vi "RP IV pattern write.vi"(4 "no bram":bool, 8 "Error In":errorcluster, 9 "Waveform parameters":T1={"Start magnitude"=1000.0, "Magnitude increment"=1000.0, "Number of pulses"=8, "Baseline length"=480, "Ramp length"=32, "Top  length"=480, "Threshold "=3000, "Processing delay"=240}, 11 "connection ID":refnum<k5>) -> (0 "Error Out":errorcluster, 3 "connection ID out":refnum<k5>, 5 "Waveform Graph":i16[](graph))   [LabVIEW 2016]
uses:
  Waform generation/Waveform parameters.ctl
  RP Command.ctl
  RP Write Command TCP.vi
panel:
  in  "Pattern":enum16{"Sine ramp", "Square"}(ring)
  out "Waveform length":u32=2048
  in  "Config offset":u64=20
  out "Step length":u32=2048
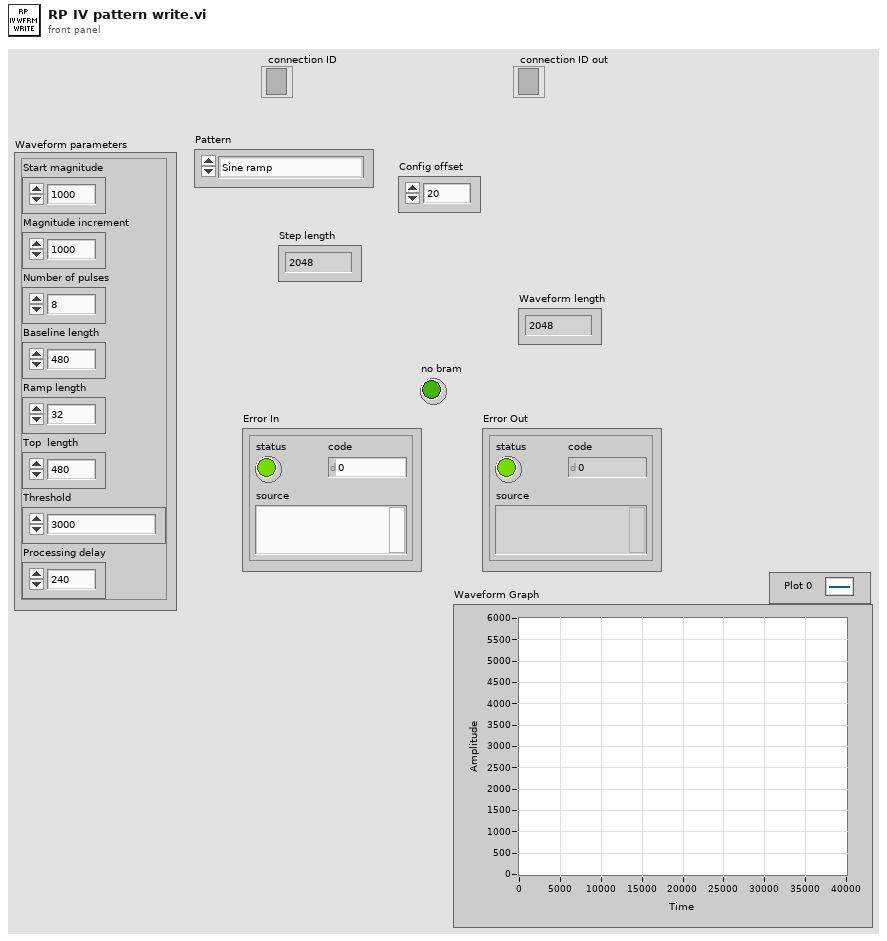
[diagram p1: front panel]
types:
  T1 = typedef "Waveform parameters.ctl" = cluster{"Start magnitude":dbl, "Magnitude increment":dbl, "Number of pulses":i32, "Baseline length":i32, "Ramp length":i32, "Top  length":i32, "Threshold ":i32, "Processing delay":u16}
  T2 = typedef "RP Command.ctl" = enum16{"Reset", "Read IDN", "Stop server", "Get status", "Get temperature", "Connect client", "Arm", "Software trigger", "Get whole buffer", "Get chunk", "System call", "Get config", "Set config", "Recieve data", "Recieve Calibartion", "Transmit data"}
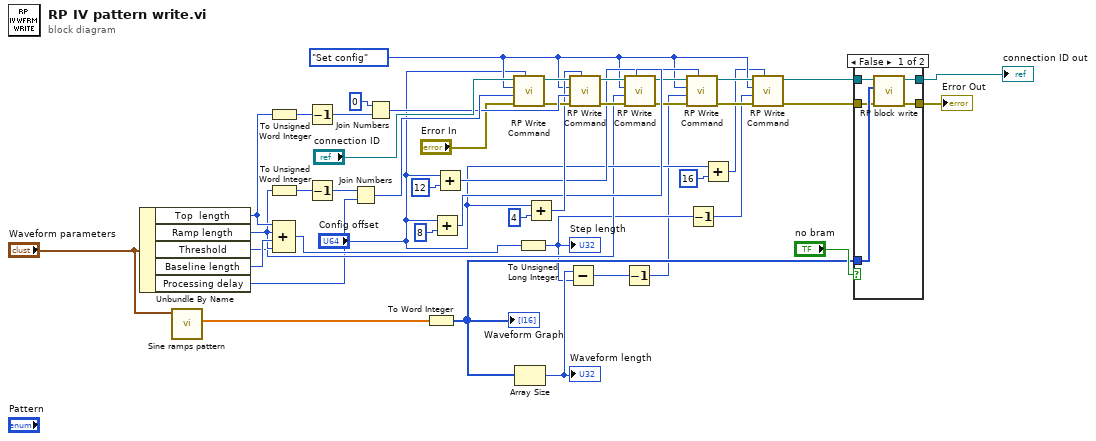
[diagram p0: block diagram]
diagram:
  w27 = RP_Command."Set config" ("Command number")
  n1 = Unbundle By Name("Waveform parameters") -> ("Top  length"=w16:i32, "Ramp length"=w14:i32, "Threshold"=w9:i32, "Baseline length"=w15:i32, "Processing delay"=w5:u16)
  n2 = call "Sine ramps pattern.vi"("Waveform parameters 2"="Waveform parameters") -> ("Waveform"=w17:dbl[])  [unwired: 8 in, 1 out]
  n3 = To Unsigned Word Integer(number=w16) -> (unsigned 16bit integer=w10:u16)
  n4 = To Unsigned Word Integer(number=w14) -> (unsigned 16bit integer=w11:u16)
  n5 = Compound Arithmetic op=ADD(w16, w14, w15, w14) -> (w7:i32)
  n6 = Decrement(x=w10) -> (x-1=w3:u16)
  n7 = Decrement(x=w11) -> (x-1=w4:u16)
  n8 = Join Numbers(hi=w4, lo=w5) -> ((hi.lo)=w45:u32)
  n9 = Join Numbers(hi=u16 0, lo=w3) -> ((hi.lo)=w42:u32)
  n10 = To Word Integer(number=w17) -> (16bit integer=w13:i16[])
  "Waveform Graph" <- w13
  n11 = Add(x="Config offset", y=u64 8) -> (x+y=w34:u64)
  n12 = Add(x="Config offset", y=u64 12) -> (x+y=w30:u64)
  n13 = call-poly "RP Write Command.vi"("Config offset"="Config offset", "Error In"="Error In", "Command payload"=w45, "Command number"=w27, "connection ID"="connection ID") -> ("Error Out"=w41:errorcluster, "connection ID out"=w44:refnum<k5>)  [unwired: 4 in, 1 out]
  n14 = Array Size(array=w13) -> (size(s)=w12:i32)
  "Waveform length" <- w12
  n15 = To Unsigned Long Integer(number=w7) -> (unsigned 32bit integer=w6:u32)
  "Step length" <- w6
  n16 = Add(x="Config offset", y=u64 4) -> (x+y=w38:u64)
  n17 = Subtract(x=w12, y=w6) -> (x-y=w8:u32)
  n18 = call-poly "RP Write Command.vi"("Config offset"=w38, "Error In"=w41, "Command payload"=w42, "Command number"=w27, "connection ID"=w44) -> ("Error Out"=w36:errorcluster, "connection ID out"=w37:refnum<k5>)  [unwired: 4 in, 1 out]
  n19 = Decrement(x=w8) -> (x-1=w2:u32)
  n20 = call-poly "RP Write Command.vi"("Config offset"=w34, "Error In"=w36, "Command payload"=w9, "Command number"=w27, "connection ID"=w37) -> ("Error Out"=w33:errorcluster, "connection ID out"=w32:refnum<k5>)  [unwired: 4 in, 1 out]
  n21 = call-poly "RP Write Command.vi"("Config offset"=w30, "Error In"=w33, "Command payload"=w2, "Command number"=w27, "connection ID"=w32) -> ("Error Out"=w29:errorcluster, "connection ID out"=w28:refnum<k5>)  [unwired: 4 in, 1 out]
  n22 = Decrement(x=w6) -> (x-1=w1:u32)
  n23 = Add(x="Config offset", y=u64 16) -> (x+y=w24:u64)
  n24 = call-poly "RP Write Command.vi"("Config offset"=w24, "Error In"=w29, "Command payload"=w1, "Command number"=w27, "connection ID"=w28) -> ("Error Out"=w22:errorcluster, "connection ID out"=w23:refnum<k5>)  [unwired: 4 in, 1 out]
  n25 = case shown="False" "no bram" {
    tunnel: w13 -> [w51 _]
    tunnel: w23 -> [w50 w53]
    tunnel: w22 -> [w49 w52]
    tunnel: [w48 w53] -> w21
    tunnel: [w47 w52] -> w20
    frame False {
      n26 = call "RP block write.vi"("Error In"=w49, "Data"=w51, "connection ID"=w50) -> ("Error Out"=w47:errorcluster, "connection ID out"=w48:refnum<k5>)  [unwired: 7 in]
    }
    frame True {
    }
  }
  "connection ID out" <- w21
  "Error Out" <- w20
